vi "Save_Measurement_data.vi"(6 "Mergedata_struct":refnum<k24>[](array[refnum]), 7 "ILSTS":refnum<k24>, 8 "错误输入（无错误）":errorcluster, 9 "Data_struct":refnum<k24>[](array[refnum])) -> (0 "错误输出":errorcluster)   [LabVIEW 2017]
doc: "Save Measurement data"
uses:
  D:/test/PDLSTS/LV_PDL_Sample/DLL/STSProcess.dll
  DLL/STSProcess.dll
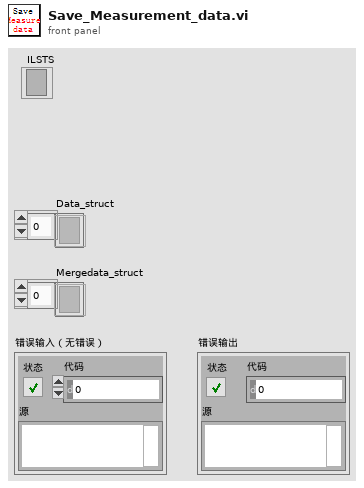
[diagram p1: front panel]
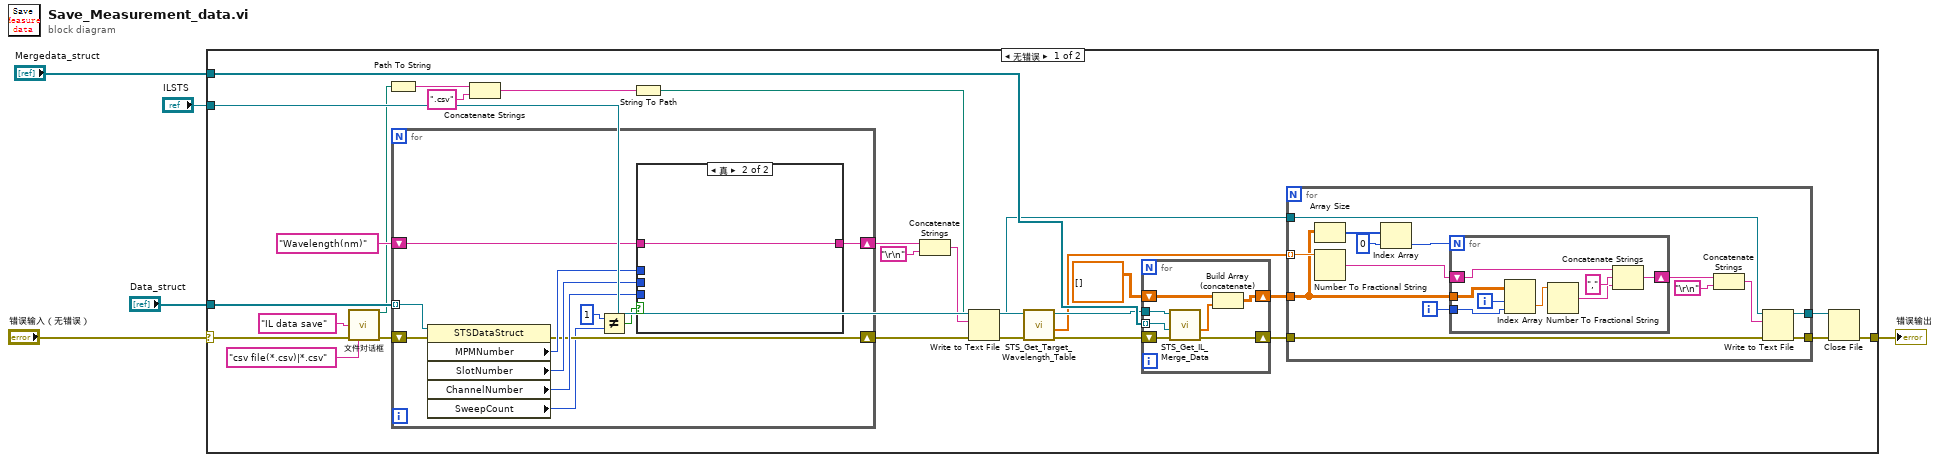
[diagram p0: block diagram]
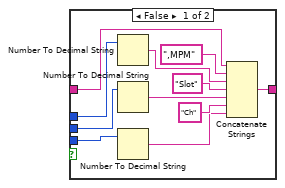
[diagram p2: hidden frame]
diagram:
  n1 = case shown="无错误" "错误输入（无错误）" {
    selector: "错误输入（无错误）" -> [w29 w86]
    tunnel: "Data_struct" -> [w21 _]
    tunnel: [w13 w86] -> w4
    tunnel: "Mergedata_struct" -> [w33 _]
    tunnel: "ILSTS" -> [w32 _]
    frame No Error {
      n2 = call "文件对话框"("default name"="IL data save" ("字符串"), "error in"=w29, "pattern (all files)"="csv file(*.csv)|*.csv") -> ("selected path"=w19:path, "error out"=w22:errorcluster)  [unwired: 9 in, 2 out]
      n3 = Path To String(path=w19) -> (string=w18:string)
      n4 = for {
        tunnel: w21 -> [w73] mode=indexing
        shift-right: [w67] -> w27
        shift-left: "Wavelength(nm)" -> [w68]
        shift-right: [w66] -> w26
        shift-left: w22 -> [w72]
        n5 = property on="属性节点" class="STSDataStruct"(reference=w73, error in=w72) -> (error out=w66:errorcluster, "MPMNumber"=w69:i32, "SlotNumber"=w70:i32, "ChannelNumber"=w71:i32, "SweepCount"=w65:i32)  [unwired: 1 out]
        n6 = Not Equal?(x=1, y=w65) -> (x != y?=w63:bool)
        n7 = case shown="真" w63 {
          tunnel: w71 -> [w84 _]
          tunnel: w70 -> [w83 _]
          tunnel: w69 -> [w82 _]
          tunnel: w68 -> [w81 w85]
          tunnel: [w74 w85] -> w67
          frame False {
            n8 = Number To Decimal String(number=w82) -> (decimal integer string=w79:string)  [unwired: 1 in]
            n9 = Number To Decimal String(number=w83) -> (decimal integer string=w77:string)  [unwired: 1 in]
            n10 = Number To Decimal String(number=w84) -> (decimal integer string=w75:string)  [unwired: 1 in]
            n11 = Concatenate Strings(w81, ",MPM" ("字符串"), w79, "Slot" ("字符串"), w77, "Ch" ("字符串"), w75) -> (w74:string)
          }
          frame True {
          }
        }
      }
      n12 = Concatenate Strings(w18, ".csv" ("名称或相对路径")) -> (w16:string)
      n13 = String To Path(string=w16) -> (path=w15:path)
      n14 = Concatenate Strings(w27, "\r\n") -> (w28:string)
      n15 = Write to Text File(file (use dialog)=w15, text=w28, error in=w26) -> (refnum out=w23:refnum<file>, error out=w20:errorcluster)  [unwired: 1 in, 1 out]
      n16 = call "STS_Get_Target_Wavelength_Table.vi"("错误输入（无错误）"=w20, ".NET引用句柄输入"=w32) -> ("error out"=w11:errorcluster, "wavelengths"=w8:dbl[], "引用输出"=w10:refnum<k24>)  [unwired: 7 in]
      n17 = for {
        tunnel: w10 -> [w61]
        tunnel: w33 -> [w60] mode=indexing
        shift-right: [w59] -> w6
        shift-left: w11 -> [w62]
        shift-right: [w56] -> w7
        shift-left: sgl[][] [] -> [w57]
        n18 = call "STS_Get_IL_Merge_Data.vi"("错误输入（无错误）"=w62, "setting"=w60, ".NET引用句柄输入"=w61) -> ("error out"=w59:errorcluster, "ilData"=w58:sgl[])  [unwired: 6 in, 1 out]
        n19 = Build Array (concatenate)(w57, w58) -> (w56:sgl[][])
      }
      n20 = for {
        tunnel: w8 -> [w47] mode=indexing
        tunnel: w7 -> [w44]
        tunnel: w6 -> [w43]
        tunnel: [w42] -> w14
        tunnel: w23 -> [w35]
        tunnel: [w34] -> w12
        i -> [w46]
        n21 = Array Size(array=w44) -> (size(s)=w38:i32[])
        n22 = Number To Fractional String(number=w47) -> (F-format string=w45:string)  [unwired: 3 in]
        n23 = Index Array(array=w38, index=0 ("索引")) -> (element=w36:i32)
        n24 = for {
          N: w36 -> [_]
          tunnel: w44 -> [w55]
          tunnel: w46 -> [w54]
          shift-right: [w50] -> w41
          shift-left: w45 -> [w51]
          i -> [w53]
          n25 = Index Array(array=w55, index (row)=w53, index (col)=w54) -> (element=w52:sgl)
          n26 = Number To Fractional String(number=w52) -> (F-format string=w48:string)  [unwired: 3 in]
          n27 = Concatenate Strings(w51, "," ("字符串"), w48) -> (w50:string)
        }
        n28 = Concatenate Strings(w41, "\r\n") -> (w39:string)
        n29 = Write to Text File(file (use dialog)=w35, text=w39, error in=w43) -> (refnum out=w34:refnum<file>, error out=w42:errorcluster)  [unwired: 1 in, 1 out]
      }
      n30 = Close File(refnum=w12, error in=w14) -> (error out=w13:errorcluster)  [unwired: 1 out]
    }
    frame Error {
    }
  }
  "错误输出" <- w4
